vi "input.vi"(8 "error in":errorcluster, 10 "data table in":T1, 11 "dds runtime in":refnum<class "dds runtime.lvclass">) -> (0 "error out":errorcluster, 2 "data table out":T1, 3 "dds runtime out":refnum<class "dds runtime.lvclass">)   [LabVIEW 2020, in "DDS runtime.lvclass"]
doc: "Provides an interface for reading data from a module at runtime. While this interface performs no operations, a child should provide an override which may read from any open sessions, references, or interfaces."
uses:
  dds runtime.lvclass
  <vilib>/NI/Tag Bus/table/data table.lvlib
  <vilib>/NI/Tag Bus/table/data polymorphs/write one/write Double.vi
  <vilib>/RTI DDS Toolkit/Library/LVDDS_library.lvlib
  <vilib>/RTI DDS Toolkit/VIs/Read_Num.vi
  <vilib>/RTI DDS Toolkit/VIs/Read_NumSgl.vi
  <vilib>/RTI DDS Toolkit/VIs/Read_NumI64.vi
  <vilib>/RTI DDS Toolkit/VIs/Read_NumI32.vi
  <vilib>/RTI DDS Toolkit/VIs/Read_NumI16.vi
  <vilib>/RTI DDS Toolkit/VIs/Read_NumI8.vi
  <vilib>/RTI DDS Toolkit/VIs/Read_NumU64.vi
  <vilib>/RTI DDS Toolkit/VIs/Read_NumU32.vi
  <vilib>/RTI DDS Toolkit/VIs/Read_NumU16.vi
  <vilib>/RTI DDS Toolkit/VIs/Read_NumU8.vi
  <vilib>/RTI DDS Toolkit/VIs/Read_Bool.vi
  <vilib>/RTI DDS Toolkit/VIs/Read_String.vi
  <vilib>/NI/Tag Bus/table/data table.ctl
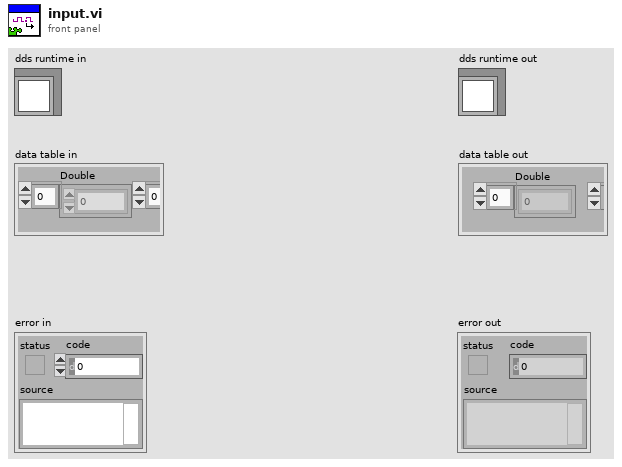
[diagram p1: front panel]
types:
  T1 = typedef "tag bus.lvlib/data table.lvlib/data table.ctl" = cluster{"Double":dbl[], "Single":sgl[], "I64":i64[], "I32":i32[], "I16":i16[], "I8":i8[], "U64":u64[], "U32":u32[], "U16":u16[], "U8":u8[], "Boolean":bool[], "String":string[], "Array of Double":cluster{"DBL Array":dbl[]}[], "Array of Single":cluster{"SGL Array":sgl[]}[], "Array of I64":cluster{"I64 Array":i64[]}[], "Array of I32":cluster{"I32 Array":i32[]}[], "Array of I16":cluster{"I16 Array":i16[]}[], "Array of I8":cluster{"I8 Array":i8[]}[], "Array of U64":cluster{"U64 Array":u64[]}[], "Array of U32":cluster{"U32 Array":u32[]}[], "Array of U16":cluster{"U16 Array":u16[]}[], "Array of U8":cluster{"U8 Array":u8[]}[], "Array of Boolean":cluster{"Boolean Array":bool[]}[], "Array of String":cluster{"String Array":string[]}[]}
  T2 = typedef "tag bus.lvlib/tag descriptor.lvclass/Data Type.ctl" = enum16{"Double", "Single", "I64", "I32", "I16", "I8", "U64", "U32", "U16", "U8", "Boolean", "String", "Array of Double", "Array of Single", "Array of I64", "Array of I32", "Array of I16", "Array of I8", "Array of U64", "Array of U32", "Array of U16", "Array of U8", "Array of Boolean", "Array of String"}
  T3 = cluster{"index":i32, "data type":T2, "ref num":u64, "new samples only":bool, "query condition":string}[]
  T4 = typedef "LVDDS_library.lvlib/DDS Sample Info.ctl" = cluster{"DDS_SampleStateKind":enum32{"DDS_INVALID_SAMPLE_STATE", "DDS_READ_SAMPLE_STATE", "DDS_NOT_READ_SAMPLE_STATE"}, "DDS_ViewStateKind":enum32{"DDS_INVALID_SAMPLE_STATE", "DDS_NEW_VIEW_STATE", "DDS_NOT_NEW_VIEW_STATE"}, "DDS_InstanceStateKind":enum32{"DDS_INVALID_STATE", "DDS_ALIVE_INSTANCE_STATE", "DDS_NOT_ALIVE_DISPOSED_INSTANCE_STATE", "", "DDS_NOT_ALIVE_NO_WRITERS_INSTANCE_STATE"}, "sec":i32, "nanosec":u32, "valid_data":bool}
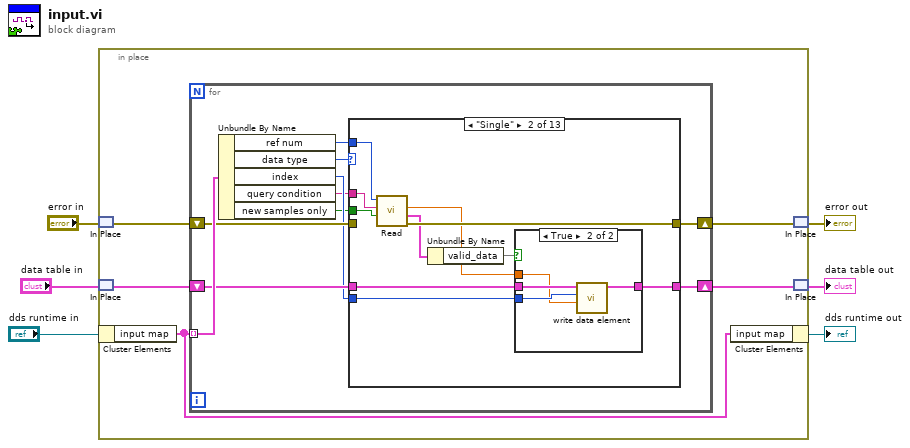
[diagram p0: block diagram]
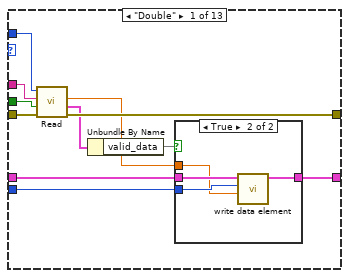
[diagram p2: hidden frame]
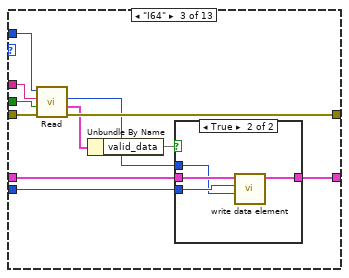
[diagram p5: hidden frame]
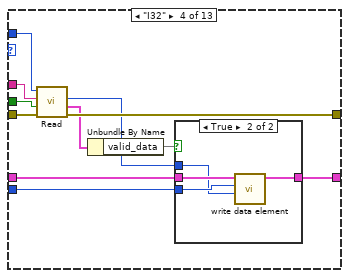
[diagram p7: hidden frame]
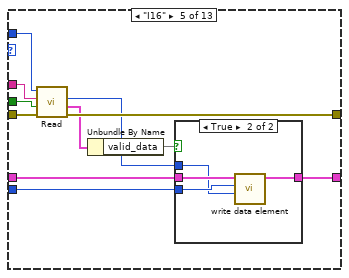
[diagram p9: hidden frame]
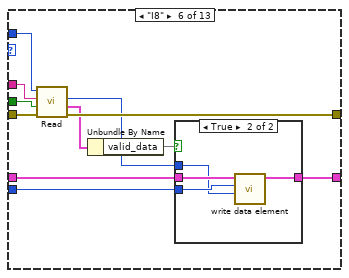
[diagram p11: hidden frame]
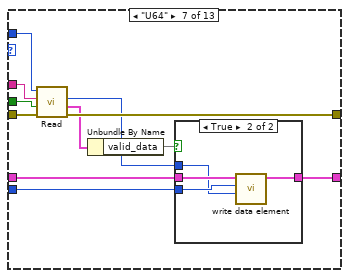
[diagram p13: hidden frame]
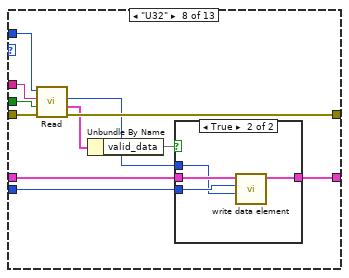
[diagram p15: hidden frame]
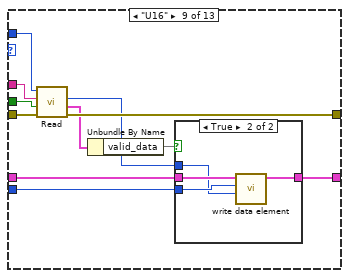
[diagram p17: hidden frame]
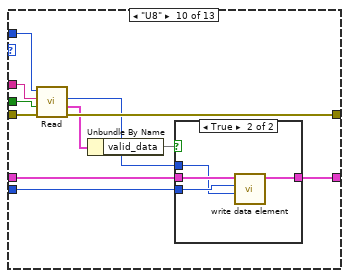
[diagram p19: hidden frame]
diagram:
  n1 = in-place {
    n2 = in-place-match #1("error in") -> (w10:errorcluster)
    n3 = in-place-match #2("data table in") -> (w11:T1)
    n4 = in-place-cluster #3("dds runtime in") -> ("input map"=w7:T3)
    n5 = for {
      tunnel: w7 -> [w21] mode=indexing
      shift-right: [w17] -> w8
      shift-left: w11 -> [w20]
      shift-right: [w18] -> w9
      shift-left: w10 -> [w19]
      n6 = Unbundle By Name(w21) -> ("ref num"=w15:u64, "data type"=w16:T2, "index"=w14:i32, "query condition"=w13:string, "new samples only"=w12:bool)
      n7 = case shown="\"Single\"" w16 {
        tunnel: w20 -> [w29 w45 w60 w76 w92 w108 w124 w140 w156 w172 w188 w204 w214]
        tunnel: w15 -> [w32 w47 w63 w79 w95 w111 w127 w143 w159 w175 w191 w207 _]
        tunnel: w19 -> [w31 _ w62 w78 w94 w110 w126 w142 w158 w174 w190 w206 w213]
        tunnel: [w30 w46 w61 w77 w93 w109 w125 w141 w157 w173 w189 w205 w213] -> w18
        tunnel: w14 -> [w28 w44 w59 w75 w91 w107 w123 w139 w155 w171 w187 w203 _]
        tunnel: [w26 w42 w57 w73 w89 w105 w121 w137 w153 w169 w185 w201 w214] -> w17
        tunnel: w13 -> [w23 w39 w54 w70 w86 w102 w118 w134 w150 w166 w182 w198 _]
        tunnel: w12 -> [w22 w38 w53 w69 w85 w101 w117 w133 w149 w165 w181 w197 _]
        frame "Double" {
          n8 = call-poly <vilib>:"Read.vi"("error in (no error)"=w31, "Only New Samples"=w22, "Query Condition"=w23, "DDS Object Ref in"=w32) -> ("error out"=w30:errorcluster, "Dds Sample Info"=w25:T4, "Data"=w27:dbl)  [unwired: 4 in, 1 out]
          n9 = Unbundle By Name(w25) -> ("valid_data"=w24)
          n10 = case shown="True" w24 {
            tunnel: w29 -> [w33 w37]
            tunnel: w28 -> [_ w35]
            tunnel: w27 -> [_ w34]
            tunnel: [w33 w36] -> w26
            frame False {
            }
            frame True {
              n11 = call-poly <vilib>:"write data element.vi"("value"=w34, "index"=w35, "data table in"=w37) -> ("data table out"=w36:T1)  [unwired: 8 in]
            }
          }
        }
        frame "Single" {
          n12 = call-poly <vilib>:"Read.vi"("Only New Samples"=w38, "Query Condition"=w39, "DDS Object Ref in"=w47) -> ("error out"=w46:errorcluster, "Dds Sample Info"=w41:T4, "Data"=w43:sgl)  [unwired: 5 in, 1 out]
          n13 = Unbundle By Name(w41) -> ("valid_data"=w40)
          n14 = case shown="True" w40 {
            tunnel: w45 -> [w48 w52]
            tunnel: w44 -> [_ w50]
            tunnel: w43 -> [_ w49]
            tunnel: [w48 w51] -> w42
            frame False {
            }
            frame True {
              n15 = call-poly <vilib>:"write data element.vi"("value"=w49, "index"=w50, "data table in"=w52) -> ("data table out"=w51:T1)  [unwired: 8 in]
            }
          }
        }
        frame "I64" {
          n16 = call-poly <vilib>:"Read.vi"("error in (no error)"=w62, "Only New Samples"=w53, "Query Condition"=w54, "DDS Object Ref in"=w63) -> ("error out"=w61:errorcluster, "Dds Sample Info"=w56:T4, "Data"=w58:i64)  [unwired: 4 in, 1 out]
          n17 = Unbundle By Name(w56) -> ("valid_data"=w55)
          n18 = case shown="True" w55 {
            tunnel: w60 -> [w64 w67]
            tunnel: w59 -> [_ w66]
            tunnel: w58 -> [_ w65]
            tunnel: [w64 w68] -> w57
            frame False {
            }
            frame True {
              n19 = call-poly <vilib>:"write data element.vi"("value"=w65, "index"=w66, "data table in"=w67) -> ("data table out"=w68:T1)  [unwired: 8 in]
            }
          }
        }
        frame "I32" {
          n20 = call-poly <vilib>:"Read.vi"("error in (no error)"=w78, "Only New Samples"=w69, "Query Condition"=w70, "DDS Object Ref in"=w79) -> ("error out"=w77:errorcluster, "Dds Sample Info"=w72:T4, "data"=w74:i32)  [unwired: 4 in, 1 out]
          n21 = Unbundle By Name(w72) -> ("valid_data"=w71)
          n22 = case shown="True" w71 {
            tunnel: w76 -> [w80 w83]
            tunnel: w75 -> [_ w82]
            tunnel: w74 -> [_ w81]
            tunnel: [w80 w84] -> w73
            frame False {
            }
            frame True {
              n23 = call-poly <vilib>:"write data element.vi"("value"=w81, "index"=w82, "data table in"=w83) -> ("data table out"=w84:T1)  [unwired: 8 in]
            }
          }
        }
        frame "I16" {
          n24 = call-poly <vilib>:"Read.vi"("error in (no error)"=w94, "Only New Samples"=w85, "Query Condition"=w86, "DDS Object Ref in"=w95) -> ("error out"=w93:errorcluster, "Dds Sample Info"=w88:T4, "Data"=w90:i16)  [unwired: 4 in, 1 out]
          n25 = Unbundle By Name(w88) -> ("valid_data"=w87)
          n26 = case shown="True" w87 {
            tunnel: w92 -> [w96 w100]
            tunnel: w91 -> [_ w98]
            tunnel: w90 -> [_ w97]
            tunnel: [w96 w99] -> w89
            frame False {
            }
            frame True {
              n27 = call-poly <vilib>:"write data element.vi"("value"=w97, "index"=w98, "data table in"=w100) -> ("data table out"=w99:T1)  [unwired: 8 in]
            }
          }
        }
        frame "I8" {
          n28 = call-poly <vilib>:"Read.vi"("error in (no error)"=w110, "Only New Samples"=w101, "Query Condition"=w102, "DDS Object Ref in"=w111) -> ("error out"=w109:errorcluster, "Dds Sample Info"=w104:T4, "Data"=w106:i8)  [unwired: 4 in, 1 out]
          n29 = Unbundle By Name(w104) -> ("valid_data"=w103)
          n30 = case shown="True" w103 {
            tunnel: w108 -> [w112 w115]
            tunnel: w107 -> [_ w114]
            tunnel: w106 -> [_ w113]
            tunnel: [w112 w116] -> w105
            frame False {
            }
            frame True {
              n31 = call-poly <vilib>:"write data element.vi"("value"=w113, "index"=w114, "data table in"=w115) -> ("data table out"=w116:T1)  [unwired: 8 in]
            }
          }
        }
        frame "U64" {
          n32 = call-poly <vilib>:"Read.vi"("error in (no error)"=w126, "Only New Samples"=w117, "Query Condition"=w118, "DDS Object Ref in"=w127) -> ("error out"=w125:errorcluster, "Dds Sample Info"=w120:T4, "Data"=w122:u64)  [unwired: 4 in, 1 out]
          n33 = Unbundle By Name(w120) -> ("valid_data"=w119)
          n34 = case shown="True" w119 {
            tunnel: w124 -> [w128 w131]
            tunnel: w123 -> [_ w130]
            tunnel: w122 -> [_ w129]
            tunnel: [w128 w132] -> w121
            frame False {
            }
            frame True {
              n35 = call-poly <vilib>:"write data element.vi"("value"=w129, "index"=w130, "data table in"=w131) -> ("data table out"=w132:T1)  [unwired: 8 in]
            }
          }
        }
        frame "U32" {
          n36 = call-poly <vilib>:"Read.vi"("error in (no error)"=w142, "Only New Samples"=w133, "Query Condition"=w134, "DDS Object Ref in"=w143) -> ("error out"=w141:errorcluster, "Dds Sample Info"=w136:T4, "Data"=w138:u32)  [unwired: 4 in, 1 out]
          n37 = Unbundle By Name(w136) -> ("valid_data"=w135)
          n38 = case shown="True" w135 {
            tunnel: w140 -> [w144 w147]
            tunnel: w139 -> [_ w146]
            tunnel: w138 -> [_ w145]
            tunnel: [w144 w148] -> w137
            frame False {
            }
            frame True {
              n39 = call-poly <vilib>:"write data element.vi"("value"=w145, "index"=w146, "data table in"=w147) -> ("data table out"=w148:T1)  [unwired: 8 in]
            }
          }
        }
        frame "U16" {
          n40 = call-poly <vilib>:"Read.vi"("error in (no error)"=w158, "Only New Samples"=w149, "Query Condition"=w150, "DDS Object Ref in"=w159) -> ("error out"=w157:errorcluster, "Dds Sample Info"=w152:T4, "Data"=w154:u16)  [unwired: 4 in, 1 out]
          n41 = Unbundle By Name(w152) -> ("valid_data"=w151)
          n42 = case shown="True" w151 {
            tunnel: w156 -> [w160 w163]
            tunnel: w155 -> [_ w162]
            tunnel: w154 -> [_ w161]
            tunnel: [w160 w164] -> w153
            frame False {
            }
            frame True {
              n43 = call-poly <vilib>:"write data element.vi"("value"=w161, "index"=w162, "data table in"=w163) -> ("data table out"=w164:T1)  [unwired: 8 in]
            }
          }
        }
        frame "U8" {
          n44 = call-poly <vilib>:"Read.vi"("error in (no error)"=w174, "Only New Samples"=w165, "Query Condition"=w166, "DDS Object Ref in"=w175) -> ("error out"=w173:errorcluster, "Dds Sample Info"=w168:T4, "Data"=w170:u8)  [unwired: 4 in, 1 out]
          n45 = Unbundle By Name(w168) -> ("valid_data"=w167)
          n46 = case shown="True" w167 {
            tunnel: w172 -> [w176 w179]
            tunnel: w171 -> [_ w178]
            tunnel: w170 -> [_ w177]
            tunnel: [w176 w180] -> w169
            frame False {
            }
            frame True {
              n47 = call-poly <vilib>:"write data element.vi"("value"=w177, "index"=w178, "data table in"=w179) -> ("data table out"=w180:T1)  [unwired: 8 in]
            }
          }
        }
        frame "Boolean" {
          n48 = call-poly <vilib>:"Read.vi"("error in (no error)"=w190, "Only New Samples"=w181, "Query Condition"=w182, "DDS Object Ref in"=w191) -> ("error out"=w189:errorcluster, "Dds Sample Info"=w184:T4, "Data"=w186:bool)  [unwired: 4 in, 1 out]
          n49 = Unbundle By Name(w184) -> ("valid_data"=w183)
          n50 = case shown="True" w183 {
            tunnel: w188 -> [w192 w195]
            tunnel: w187 -> [_ w194]
            tunnel: w186 -> [_ w193]
            tunnel: [w192 w196] -> w185
            frame False {
            }
            frame True {
              n51 = call-poly <vilib>:"write data element.vi"("value"=w193, "index"=w194, "data table in"=w195) -> ("data table out"=w196:T1)  [unwired: 8 in]
            }
          }
        }
        frame "String" {
          n52 = call-poly <vilib>:"Read.vi"("error in (no error)"=w206, "Only New Samples"=w197, "Query Condition"=w198, "DDS Object Ref in"=w207) -> ("error out"=w205:errorcluster, "Dds Sample Info"=w200:T4, "Data"=w202:string)  [unwired: 4 in, 1 out]
          n53 = Unbundle By Name(w200) -> ("valid_data"=w199)
          n54 = case shown="True" w199 {
            tunnel: w204 -> [w208 w212]
            tunnel: w203 -> [_ w210]
            tunnel: w202 -> [_ w209]
            tunnel: [w208 w211] -> w201
            frame False {
            }
            frame True {
              n55 = call-poly <vilib>:"write data element.vi"("value"=w209, "index"=w210, "data table in"=w212) -> ("data table out"=w211:T1)  [unwired: 8 in]
            }
          }
        }
        frame Default {
          # "#TODO\nThis case should never be reached.\nThrow error."
        }
      }
    }
    n56 = in-place-cluster #3("input map"=w7) -> (→"dds runtime out":refnum<class "dds runtime.lvclass">)
    n57 = in-place-match #1(w9) -> (→"error out":errorcluster)
    n58 = in-place-match #2(w8) -> (→"data table out":T1)
  }
